vi "Create.vi"(10 "Entity ID":T1) -> (3 "ID out":refnum<class "ID.lvclass">)   [LabVIEW 2022 SP3, in "Conditum.lvlib" / "Columns.lvlib" / "ID.lvclass"]
uses:
  ID.lvclass
  ID.lvclass/ID.ctl
  Entity ID.ctl
  Conditum.lvlib
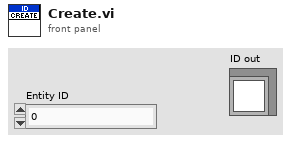
[diagram p1: front panel]
types:
  T1 = typedef "Conditum.lvlib/Entity ID.ctl" = i64
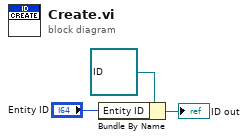
[diagram p0: block diagram]
diagram:
  n1 = Bundle By Name(cluster=refnum<class "ID.lvclass"> refnum ("ID out"), "Entity ID"="Entity ID") -> (→"ID out":refnum<class "ID.lvclass">)
